vi "CreateMessageQueues.vi"(5 "elements to preallocate per priority (0)":i32, 6 "create if not found? (T)":bool=TRUE, 7 "max queue size per priority (-1, unlimited)":i32=-1, 8 "error in":errorcluster, 10 "number of priorities":i32=3, 11 "name (\"\", unnamed)":string) -> (0 "error out":errorcluster, 1 "total elements preallocated":i32, 2 "number of priorities used":i32, 3 "queues out":refnum<class "CLM_PriorityLocalMessage.lvclass">, 4 "created new?":bool)   [LabVIEW 2013, in "CLM_PriorityLocalMessage.lvclass"]
uses:
  CLM_PriorityLocalMessage.lvclass
  FG_NamedQueuesAction.ctl
  LocalMessage_Queue/CLM_LocalMessage_Queue.lvclass/CLM_LocalMessage_Queue.ctl
  CLM_PriorityLocalMessage.lvclass/CLM_PriorityLocalMessage.ctl
  LocalMessage_Queue/SendMultipleQueueMessages.vi
  LocalMessage_Queue/FlushQueueMessage.vi
  LocalMessage_Queue/SendQueueMessage.vi
  LocalMessage_Queue/SendQueueMessage_Cluster.vi
  LocalMessage/BundleMessageCluster.vi
  <vilib>/Utility/error.llb/Clear Errors.vi
  LocalMessage_Queue/CLM_LocalMessage_Queue.lvclass
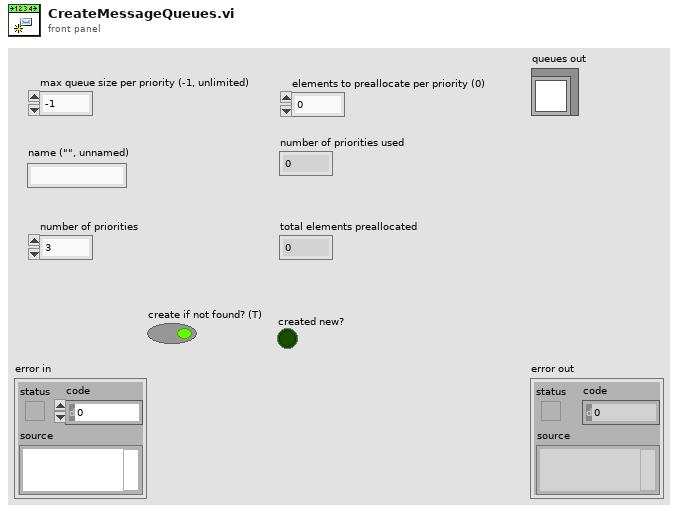
[diagram p1: front panel]
types:
  T1 = typedef "CLM_PriorityLocalMessage.lvclass/FG_NamedQueuesAction.ctl" = enum16{"Get", "Add", "Remove", "RemoveAll"}
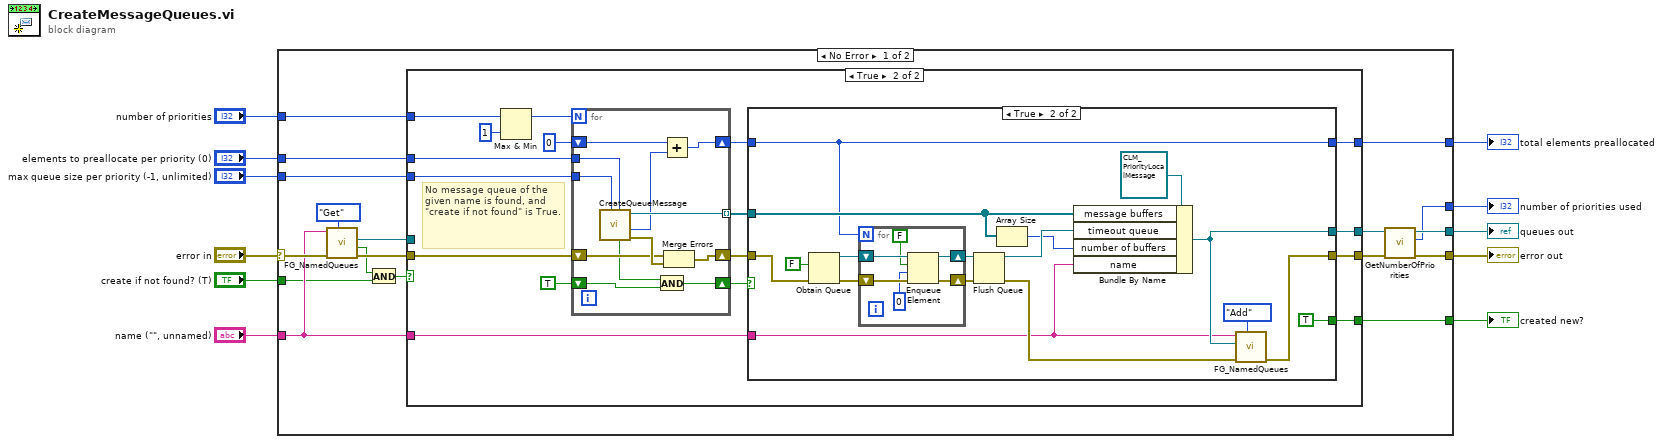
[diagram p0: block diagram]
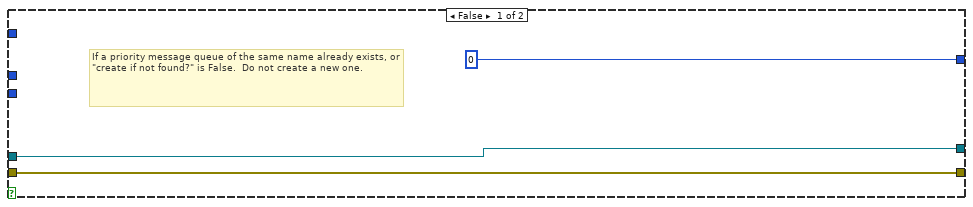
[diagram p2: hidden frame]
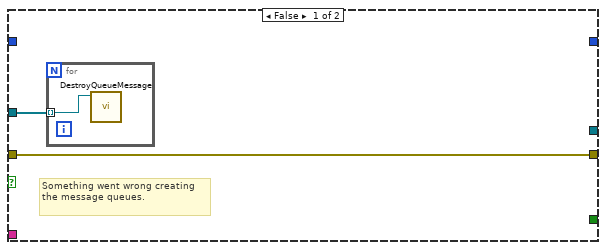
[diagram p3: hidden frame]
diagram:
  n1 = case shown="No Error" "error in" {
    selector: "error in" -> [w25 w88]
    tunnel: [w20 w88] -> w10
    tunnel: "number of priorities" -> [w29 _]
    tunnel: "max queue size per priority (-1, unlimited)" -> [w27 _]
    tunnel: "elements to preallocate per priority (0)" -> [w28 _]
    tunnel: [w22 _] -> w6
    tunnel: [w19 _] -> w5
    tunnel: [w26 _] -> w4
    tunnel: "name (\"\", unnamed)" -> [w17 _]
    tunnel: [w16 _] -> w2
    tunnel: "create if not found? (T)" -> [w14 _]
    frame No Error {
      n2 = call "FG_NamedQueues.vi"("action"=FG_NamedQueuesAction."Get", "error in"=w25, "name"=w17) -> ("error out"=w24:errorcluster, "failed?"=w13:bool, "queues out"=w18:refnum<class "CLM_PriorityLocalMessage.lvclass">)  [unwired: 6 in]
      n3 = And(x=w13, y=w14) -> (x .and. y?=w12:bool)
      n4 = case shown="True" w12 {
        tunnel: w29 -> [_ w49]
        tunnel: w28 -> [_ w47]
        tunnel: w27 -> [_ w46]
        tunnel: [0 w33] -> w26
        tunnel: w24 -> [w32 w40]
        tunnel: [w31 w39] -> w23
        tunnel: [w32 w38] -> w21
        tunnel: w18 -> [w31 _]
        tunnel: w17 -> [_ w37]
        tunnel: [_ w36] -> w16
        frame False {
          # "If a priority message queue of the same name already exists, or \"create if not found?\" is False.  Do not create a new one."
        }
        frame True {
          # "No message queue of the given name is found, and \"create if not found\" is True."
          n5 = Max & Min(x=w49, y=1) -> (max(x,y)=w41:i32)  [unwired: 1 out]
          n6 = for {
            N: w41 -> [_]
            tunnel: w47 -> [w86]
            tunnel: w46 -> [w87]
            tunnel: [w85] -> w42 mode=indexing
            shift-right: [w83] -> w45
            shift-left: w40 -> [w82]
            shift-right: [w80] -> w43
            shift-left: 0 -> [w79]
            shift-right: [w77] -> w34
            shift-left: TRUE -> [w76]
            n7 = call "CreateQueueMessage.vi"("elements to preallocate (0)"=w86, "max queue size (-1, unlimited)"=w87) -> ("error out"=w84:errorcluster, "elements preallocated"=w81:i32, "message ref"=w85:refnum<class "CLM_LocalMessage_Queue.lvclass">, "created new?"=w78:bool)  [unwired: 6 in]
            n8 = And(x=w78, y=w76) -> (x .and. y?=w77:bool)
            n9 = Add(x=w79, y=w81) -> (x+y=w80:i32)
            n10 = Merge Errors(w82, w84) -> (w83:errorcluster)
          }
          n11 = case shown="True" w34 {
            tunnel: w45 -> [w51 w67]
            tunnel: w43 -> [_ w53]
            tunnel: w42 -> [w50 w61]
            tunnel: [_ w58] -> w39
            tunnel: [w51 w56] -> w38
            tunnel: w37 -> [_ w55]
            tunnel: [_ TRUE] -> w36
            tunnel: [_ w53] -> w33
            frame False {
              # "Something went wrong creating the message queues."
              n12 = for {
                tunnel: w50 -> [w52] mode=indexing
                n13 = call "DestroyQueueMessage.vi"("message ref in"=w52) -> ()  [unwired: 9 in, 2 out]
              }
            }
            frame True {
              n14 = Obtain Queue(element data type=FALSE, error in (no error)=w67) -> (queue out=w66:refnum<queue>, error out=w65:errorcluster)  [unwired: 3 in, 1 out]
              n15 = for {
                N: w53 -> [_]
                shift-right: [w72] -> w63
                shift-left: w66 -> [w75]
                shift-right: [w73] -> w64
                shift-left: w65 -> [w74]
                n16 = Enqueue Element(queue=w75, element=FALSE, timeout in ms (-1)=0, error in (no error)=w74) -> (queue out=w72:refnum<queue>, error out=w73:errorcluster)  [unwired: 1 out]
              }
              n17 = Flush Queue(queue=w63, error in (no error)=w64) -> (queue out=w62:refnum<queue>, error out=w57:errorcluster)  [unwired: 1 out]
              n18 = Array Size(array=w61) -> (size(s)=w60:i32)
              n19 = Bundle By Name(cluster=refnum<class "CLM_PriorityLocalMessage.lvclass"> refnum ("NISE_PriorityLocalMessage.lvclass"), "message buffers"=w61, "timeout queue"=w62, "number of buffers"=w60, "name"=w55) -> (w58:refnum<class "CLM_PriorityLocalMessage.lvclass">)
              n20 = call "FG_NamedQueues.vi"("action"=FG_NamedQueuesAction."Add", "error in"=w57, "queues in"=w58, "name"=w55) -> ("error out"=w56:errorcluster)  [unwired: 5 in, 2 out]
            }
          }
        }
      }
      n21 = call "GetNumberOfPriorities.vi"("error in"=w21, "queues in"=w23) -> ("error out"=w20:errorcluster, "number of priorities"=w19:i32, "queues out"=w22:refnum<class "CLM_PriorityLocalMessage.lvclass">)  [unwired: 7 in]
    }
    frame Error {
    }
  }
  "error out" <- w10
  "queues out" <- w6
  "number of priorities used" <- w5
  "total elements preallocated" <- w4
  "created new?" <- w2
